vi "10 - Design Pattern - When Generation Rate exceeds Handling Rate (Dropped Frames).vi"() -> ()   [LabVIEW 2012]
uses:
  <vilib>/ptbypt/NI_PtbyPt.lvlib
panel:
  out "Handled Signal":cluster{"X":dbl, "Y":dbl}[](graph)
  out "Fraction of Dropped Events":dbl(graph)
  out "Handled":i32
  out "Dropped":i32
  out "Published":i32
  out "Events/sec":dbl caption="Publisher Rate" format="%.0f events/sec"
  in  "Throttler Period":u32(ring) caption="Handler Throttle" items=["None"=0, "50msec"=50, "200msec"=200, "500msec"=500, "1000msec"=1000]
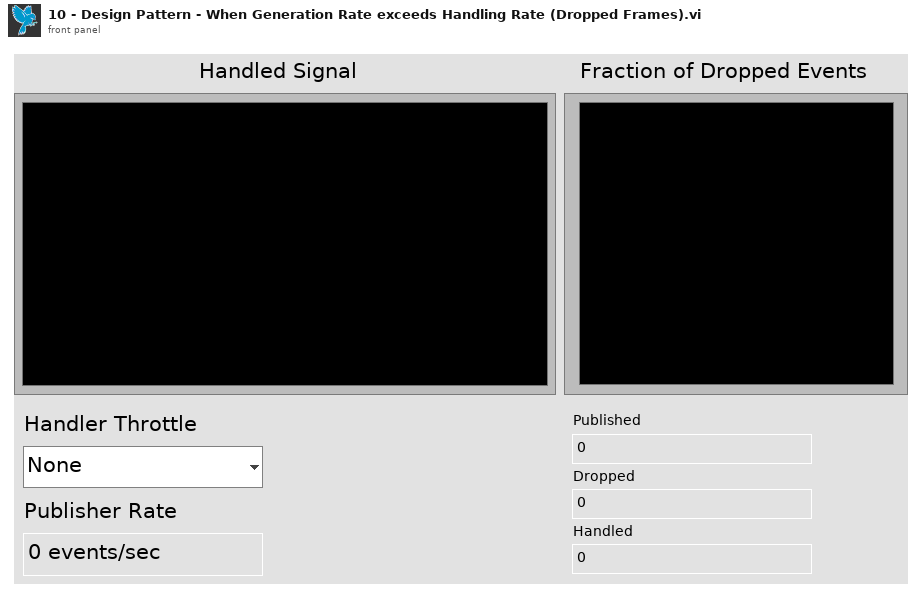
[diagram p1: front panel]
types:
  T1 = cluster{"millisecond timer value":u32, "sine wave":dbl}
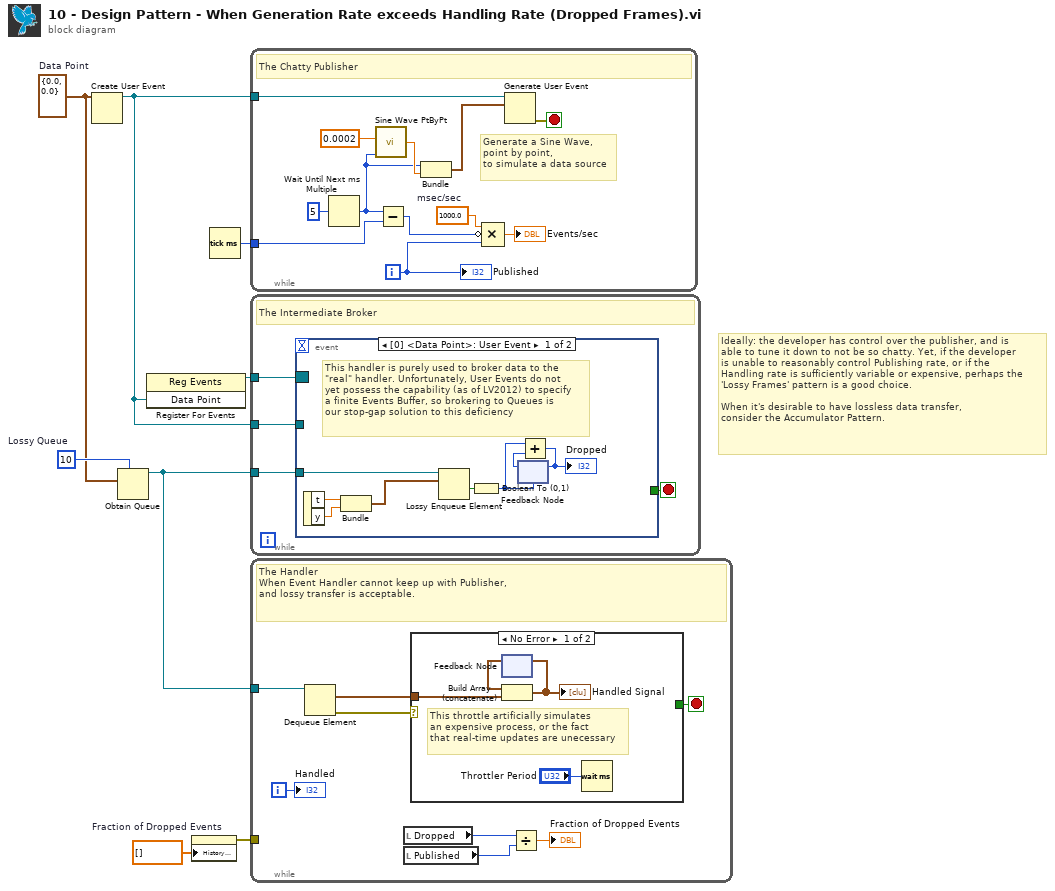
[diagram p0: block diagram]
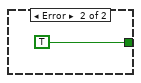
[diagram p2: hidden frame]
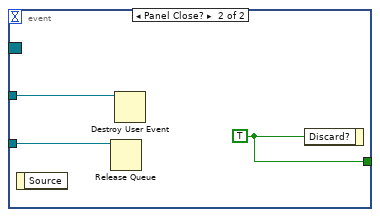
[diagram p3: hidden frame]
diagram:
  w3 = cluster{"t":dbl, "y":dbl} {"t"=0.0, "y"=0.0}  # Data Point
  w8 = 10  # Lossy Queue
  # "Ideally: the developer has control over the publisher, and is\nable to tune it down to not be so chatty. Yet, if the developer\nis unable to reasonably control Publishing rate, or if the\nHandling rate is sufficiently variable or expensive, perhaps the\n'Lossy Frames' pattern is a good choice.\n\nWhen it's desirable to have lossless data transfer,\nconsider the Accumulator Pattern."
  n1 = Create User Event(user event datatype=w3) -> (user event=w4:refnum<user-event>)  [unwired: 1 in, 1 out]
  n2 = Obtain Queue(max queue size (-1, unlimited)=w8, element data type=w3) -> (queue out=w7:refnum<queue>)  [unwired: 3 in, 2 out]
  n3 = register-events(w4) -> (reference out=w5:refnum<event-registration>)  [unwired: 2 in, 1 out]
  n4 = property on="Fraction of Dropped Events" class="WFChart (strict)"("History Data"=dbl[] []) -> (error out=w1:errorcluster)  [unwired: 2 in, 1 out]
  n5 = Tick Count (ms)() -> (millisecond timer value=w6:u32)
  n6 = while {
    tunnel: w4 -> [w20]
    tunnel: w6 -> [w18]
    i -> [w9]
    stop <- w19 stop-if-true
    w17 = 1000.0  # msec/sec
    # "Generate a Sine Wave,\npoint by point,\nto simulate a data source"
    # "The Chatty Publisher"
    n7 = Wait Until Next ms Multiple(millisecond multiple=u32 5 ("milliseconds to wait")) -> (millisecond timer value=w11:u32)
    n8 = call <vilib>:"Sine Wave PtByPt.vi"("time"=w11, "frequency"=0.0002) -> ("sine wave"=w12:dbl)  [unwired: 2 in]
    n9 = Subtract(x=w11, y=w18) -> (x-y=w16:u32)
    n10 = Bundle("millisecond timer value"=w11, "sine wave"=w12) -> (w10:T1)  [unwired: 1 in]
    n11 = Compound Arithmetic op=MULTIPLY(w17, invert w16, w9) -> (→"Events/sec":dbl)
    n12 = Generate User Event(user event=w20, event data cluster=w10) -> (error out=w19:errorcluster)  [unwired: 1 in, 1 out]
    "Published" <- w9
  }
  n13 = while {
    tunnel: w7 -> [w23]
    tunnel: w5 -> [w22]
    tunnel: w4 -> [w21]
    stop <- w24 stop-if-true
    # "The Intermediate Broker"
    n14 = event shown="[0] <Data Point>: User Event" {
      selector: w22 -> [_ _]
      dyn-events: _ -> [_ _]
      timeout: _ -> [_ _]
      tunnel: [_ w35] -> w24
      tunnel: w23 -> [w32 w34]
      tunnel: w21 -> [_ w33]
      event User Event {
        # "This handler is purely used to broker data to the\n\"real\" handler. Unfortunately, User Events do not\nyet possess the capability (as of LV2012) to specify\na finite Events Buffer, so brokering to Queues is\nour stop-gap solution to this deficiency"
        n15 = event-data() -> ("t"=w31:dbl, "y"=w30:dbl)  [unwired: 1 in]
        n16 = Bundle("t"=w31, "y"=w30) -> (w29:cluster{"t":dbl, "y":dbl})  [unwired: 1 in]
        n17 = Lossy Enqueue Element(queue=w32, element=w29) -> (overflow?=w28:bool)  [unwired: 1 in, 3 out]
        n18 = Boolean To (0,1)(Boolean=w28) -> (0, 1=w25:i16)
        n19 = feedback #1(w25) -> (w26:i16)
        n20 = Add(x=w25, y=w26) -> (x+y=w27:i16)
        "Dropped" <- w27
        n21 = feedback-in #1(w27) -> ()
      }
      event Panel Close? {
        w35 = TRUE ("Discard?")
        n22 = event-data() -> ()  [unwired: 1 in, 1 out]
        n23 = Release Queue(queue=w34) -> ()  [unwired: 2 in, 3 out]
        n24 = Destroy User Event(user event=w33) -> ()  [unwired: 1 in, 1 out]
        n25 = event-data("Discard?"=w35) -> ()  [unwired: 1 in, 1 out]
      }
    }
  }
  n26 = while {
    tunnel: w7 -> [w43]
    tunnel: w1 -> [_]
    i -> [w39]
    stop <- w40 stop-if-true
    # "The Handler\nWhen Event Handler cannot keep up with Publisher,\nand lossy transfer is acceptable."
    n27 = Dequeue Element(queue=w43) -> (element=w41:cluster{"t":dbl, "y":dbl}, error out=w42:errorcluster)  [unwired: 2 in, 2 out]
    n28 = local read "Dropped"() -> (w38:i32)
    n29 = local read "Published"() -> (w37:i32)
    n30 = case shown="No Error" w42 {
      tunnel: w41 -> [w46 _]
      tunnel: [_ TRUE] -> w40
      frame No Error {
        # "This throttle artificially simulates\nan expensive process, or the fact\nthat real-time updates are unecessary"
        n31 = feedback #2() -> (w45:cluster{"t":dbl, "y":dbl}[])  [unwired: 1 in]
        n32 = Build Array (concatenate)(w45, w46) -> (w44:cluster{"t":dbl, "y":dbl}[])
        "Handled Signal" <- w44
        n33 = feedback-in #2(w44) -> ()
        n34 = Wait (ms)(milliseconds to wait="Throttler Period") -> ()  [unwired: 1 out]
      }
      frame Error {
      }
    }
    n35 = Divide(x=w38, y=w37) -> (x/y=→"Fraction of Dropped Events":dbl)
    "Handled" <- w39
  }
